vi "Get MSS.vi"(11 "Task Actor in":refnum<class "Task Actor.lvclass">) -> (2 "Measure and Stimulus Subsystems.lvclass":refnum<class "Measure and Stimulus Subsystems.lvclass">, 3 "Task Actor out":refnum<class "Task Actor.lvclass">)   [LabVIEW 2023, in "Task Actor.lvlib" / "Task Actor.lvclass"]
uses:
  Task Actor.lvclass
  Measure and Stimulus Subsystems/Measure and Stimulus Subsystems.lvclass
  Task Actor.lvclass/Task Actor.ctl
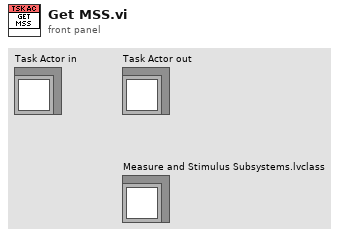
[diagram p1: front panel]
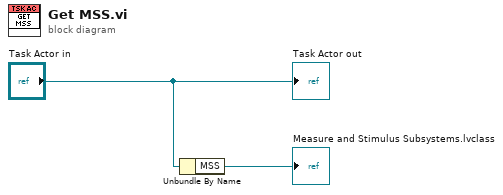
[diagram p0: block diagram]
diagram:
  n1 = Unbundle By Name("Task Actor in") -> ("MSS"=→"Measure and Stimulus Subsystems.lvclass":refnum<class "Measure and Stimulus Subsystems.lvclass">)
  "Task Actor out" <- "Task Actor in"
